vi "Outlier_Test.vi"() -> ()   [LabVIEW 2013]
uses:
  Grubbs_Test_States.ctl
  <vilib>/Utility/file.llb/Read From Spreadsheet File (DBL).vi
  <vilib>/Analysis/NI_AALBase.lvlib
panel:
  in  "Grubs":bool=TRUE
  out "Обработанные результаты":dbl[](graph)
  out "Исходная выборка":dbl[](graph)
  out "СКО":dbl
  out "Среднее":dbl
  out "Array":dbl[](array[numeric])
  in  "Уровень значимости":dbl
  in  "Путь к файлу данных":path
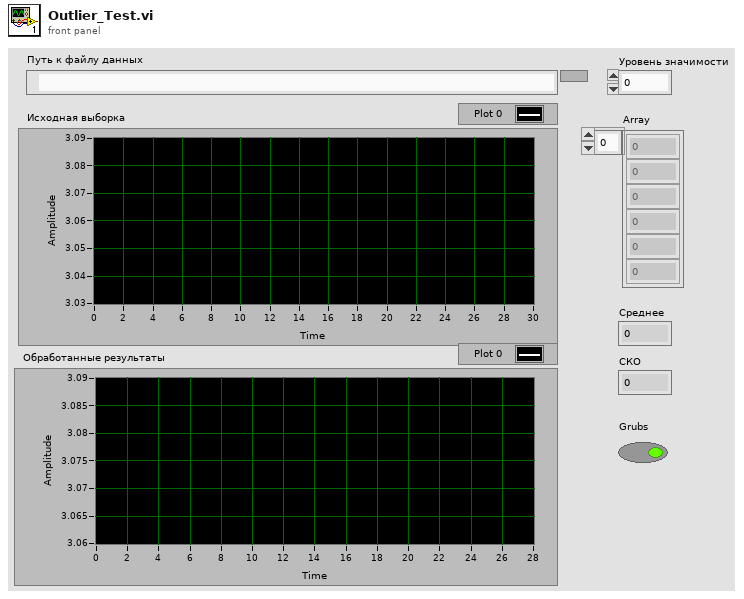
[diagram p1: front panel]
types:
  T1 = typedef "Grubbs_Test_States.ctl" = enum16{"Инициализация", "Расчет ошибок", "Проверка на промахи", "Завершение работы"}
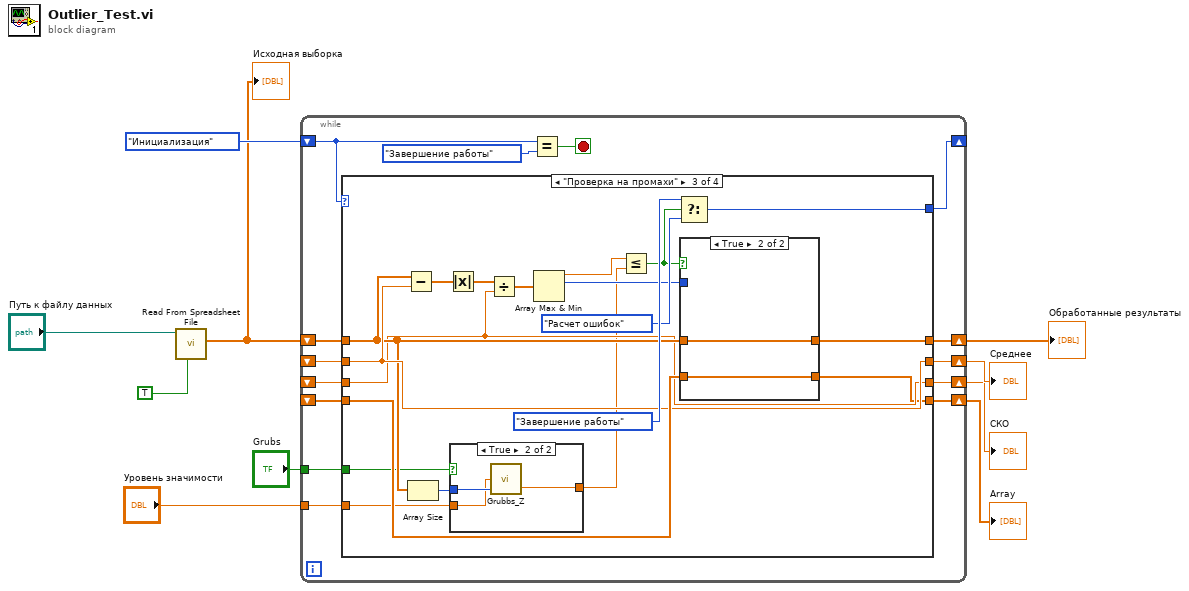
[diagram p0: block diagram]
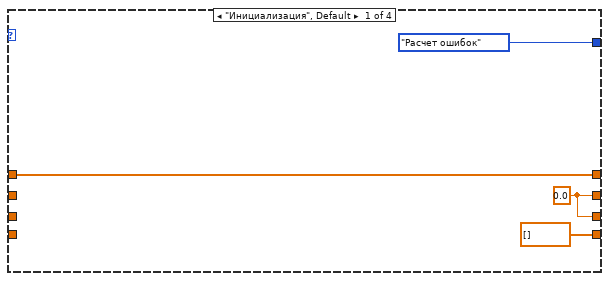
[diagram p2: hidden frame]
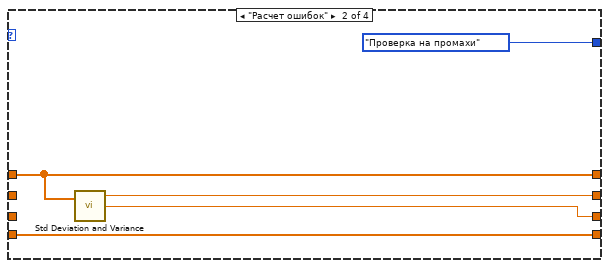
[diagram p3: hidden frame]
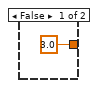
[diagram p4: hidden frame]
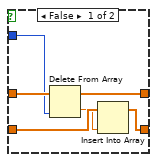
[diagram p5: hidden frame]
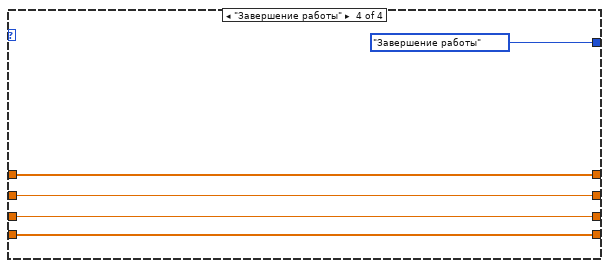
[diagram p6: hidden frame]
diagram:
  n1 = call-poly <vilib>:"Read From Spreadsheet File.vi"("transpose (no:F)"=TRUE, "file path (dialog if empty)"="Путь к файлу данных") -> ("first row"=w4:dbl[])  [unwired: 5 in, 4 out]
  "Исходная выборка" <- w4
  n2 = while {
    shift-right: [w24] -> _
    shift-left: Grubbs_Test_States."Инициализация" -> [w22]
    shift-right: [w17] -> w3
    shift-left: w4 -> [w18]
    shift-right: [w12] -> w9
    shift-left: _ -> [w14]
    shift-right: [w20] -> w8
    shift-left: _ -> [w13]
    shift-right: [w16] -> w2
    shift-left: _ -> [w15]
    tunnel: "Уровень значимости" -> [w19]
    tunnel: "Grubs" -> [w11]
    stop <- w21 stop-if-true
    n3 = case shown="\"Проверка на промахи\"" w22 {
      tunnel: [Grubbs_Test_States."Расчет ошибок" Grubbs_Test_States."Проверка на промахи" w48 Grubbs_Test_States."Завершение работы"] -> w24
      tunnel: [w27 w30 w43 w67] -> w20
      tunnel: w19 -> [_ _ w36 _]
      tunnel: [w26 w32 w39 w69] -> w17
      tunnel: w18 -> [w26 w32 w44 w69]
      tunnel: [dbl[] [] w33 w38 w66] -> w16
      tunnel: w15 -> [_ w33 w52 w66]
      tunnel: w14 -> [_ _ w45 w68]
      tunnel: w13 -> [_ _ w43 w67]
      tunnel: [w27 w31 w45 w68] -> w12
      tunnel: w11 -> [_ _ w34 _]
      frame "Инициализация", Default {
        w27 = 0.0
      }
      frame "Расчет ошибок" {
        n4 = call <vilib>:"Std Deviation and Variance.vi"("X"=w32) -> ("mean"=w31:dbl, "standard deviation"=w30:dbl)  [unwired: 1 in, 1 out]
      }
      frame "Проверка на промахи" {
        n5 = Subtract(x=w44, y=w45) -> (x-y=w46:dbl[])
        n6 = Array Size(array=w44) -> (size(s)=w37:i32)
        n7 = Absolute Value(x=w46) -> (abs(x)=w51:dbl[])
        n8 = case shown="True" w34 {
          tunnel: w37 -> [_ w56]
          tunnel: w36 -> [_ w55]
          tunnel: [3.0 w54] -> w35
          frame False {
          }
          frame True {
            n9 = call "Grubbs_Z.vi"("n"=w56, "q"=w55) -> ("G"=w54:dbl)  [unwired: 2 in]
          }
        }
        n10 = Divide(x=w51, y=w43) -> (x/y=w42:dbl[])
        n11 = Array Max & Min(array=w42) -> (max value=w41:dbl, max index (indices)=w40:i32)  [unwired: 2 out]
        n12 = Less Or Equal?(x=w41, y=w35) -> (x <= y?=w47:bool)
        n13 = Select(t=Grubbs_Test_States."Завершение работы", s=w47, f=Grubbs_Test_States."Расчет ошибок") -> (s? t:f=w48:T1)
        n14 = case shown="True" w47 {
          tunnel: w44 -> [w62 w64]
          tunnel: [w61 w64] -> w39
          tunnel: w52 -> [w60 w63]
          tunnel: [w59 w63] -> w38
          tunnel: w40 -> [w57 _]
          frame False {
            n15 = Delete From Array(array=w62, index=w57) -> (deleted portion=w58:dbl, array with subset deleted=w61:dbl[])  [unwired: 1 in]
            n16 = Insert Into Array(array=w60, new element=w58) -> (w59:dbl[])  [unwired: 1 in]
          }
          frame True {
          }
        }
      }
      frame "Завершение работы" {
      }
    }
    n17 = Equal?(x=w22, y=Grubbs_Test_States."Завершение работы") -> (x = y?=w21:bool)
  }
  "Array" <- w2
  "Среднее" <- w9
  "СКО" <- w8
  "Обработанные результаты" <- w3
